vi "HolonomicController_Example.vi"(6 "EnableClosedLoop":bool=TRUE, 7 "Orientation Dmd In":dbl, 8 "Init":bool=TRUE, 9 "Reverse":bool, 10 "Follow Orientation":bool) -> (0 "AtReference":bool, 3 "Chassis Velocity Target":T2 {"vOmega" format="%10.3f"; "vY" format="%10.3f"; "vX" format="%10.3f"}, 4 "Time Offset":dbl=-1.0 format="%16.4f", 5 "Orientation Target":dbl, 11 "Gyro Heading":dbl)   [LabVIEW 2019]
uses:
  <vilib>/Rock Robotics/WPI/ThirdParty/JAS_Junk/TrajLib/TypeDef/CHASSIS_SPEEDS.ctl
  <vilib>/Rock Robotics/WPI/ThirdParty/JAS_Junk/TrajLib/TypeDef/TRAJ_STATE.ctl
  <vilib>/Rock Robotics/WPI/ThirdParty/JAS_Junk/TrajLib/TypeDef/POSE2D.ctl
  <vilib>/Rock Robotics/WPI/ThirdParty/JAS_Junk/TrajLib/TypeDef/TRANSLATION2D.ctl
  <vilib>/Rock Robotics/WPI/ThirdParty/JAS_Junk/TrajLib/TypeDef/ROTATION2D.ctl
  <vilib>/Rock Robotics/WPI/ThirdParty/JAS_Junk/TrajLib/MedianFilter_New.vi
  <vilib>/Rock Robotics/WPI/ThirdParty/JAS_Junk/TrajLib/MedianFilter_ResetToValue.vi
  SubVI/HOL_Robot Global Data.vi
  <vilib>/Rock Robotics/WPI/ThirdParty/JAS_Junk/TrajLib/MedianFilter_Calculate.vi
  <vilib>/Rock Robotics/WPI/ThirdParty/JAS_Junk/TrajLib/Trajectory_Library.lvlib
panel:
  in  "Tab Control":T1(tab)
  out "OutputTRAJ_STATE":T3={"TimeSeconds"=0.0, "Velocity"=0.0, "Acceleration"=0.0, "POSE"={"TRANSLATION"={"X"=0.0, "Y"=0.0}, "ROTATION"={"VALUE"=0.0, "COS"=1.0, "SIN"=0.0}}, "Curvature"=0.0} {"POSE"."ROTATION"."SIN" format="%13.4f"; "POSE"."ROTATION"."COS" format="%13.4f"; "POSE"."ROTATION"."VALUE" format="%13.4f"; "POSE"."TRANSLATION"."Y" format="%14.3f"; "POSE"."TRANSLATION"."X" format="%14.3f"}
  in  "Step":bool
  in  "Trajectory File Name":path=path "Sample-Robot-2-Trajectory-TrajLibrary.csv"
  out "Traj File Good":bool
  out "Module Ang\nRadians":dbl
  out "Module Speed\nM/S":dbl
  in  "Run":bool
  out "Rel Odom":T4={"TRANSLATION"={"X"=0.0, "Y"=0.0}, "ROTATION"={"VALUE"=0.0, "COS"=1.0, "SIN"=0.0}} {"ROTATION"."SIN" format="%13.4f"; "ROTATION"."COS" format="%13.4f"; "ROTATION"."VALUE" format="%13.4f"; "TRANSLATION"."Y" format="%14.3f"; "TRANSLATION"."X" format="%14.3f"}
  out "Error and Corr":T7 {"Error Pose"."ROTATION"."SIN" format="%13.4f"; "Error Pose"."ROTATION"."COS" format="%13.4f"; "Error Pose"."ROTATION"."VALUE" format="%13.4f"; "Error Pose"."TRANSLATION"."Y" format="%14.3f"; "Error Pose"."TRANSLATION"."X" format="%14.3f"}
  out "Abs Odom":T4={"TRANSLATION"={"X"=0.0, "Y"=0.0}, "ROTATION"={"VALUE"=0.0, "COS"=1.0, "SIN"=0.0}} {"ROTATION"."SIN" format="%13.4f"; "ROTATION"."COS" format="%13.4f"; "ROTATION"."VALUE" format="%13.4f"; "TRANSLATION"."Y" format="%14.3f"; "TRANSLATION"."X" format="%14.3f"}
  out "Traj Err":cluster{"X":dbl, "Y":dbl, "Angle":dbl}(graph)
  out "ChasisSpeedOutput":cluster{"vX":dbl, "vY":dbl, "vOmega":dbl}(graph)
  out "Robot Position":cluster{dbl[], dbl[]}[](graph)
  # "Module States"
  # "For now all modules use this value..."
  # "(FOR TESTING)"
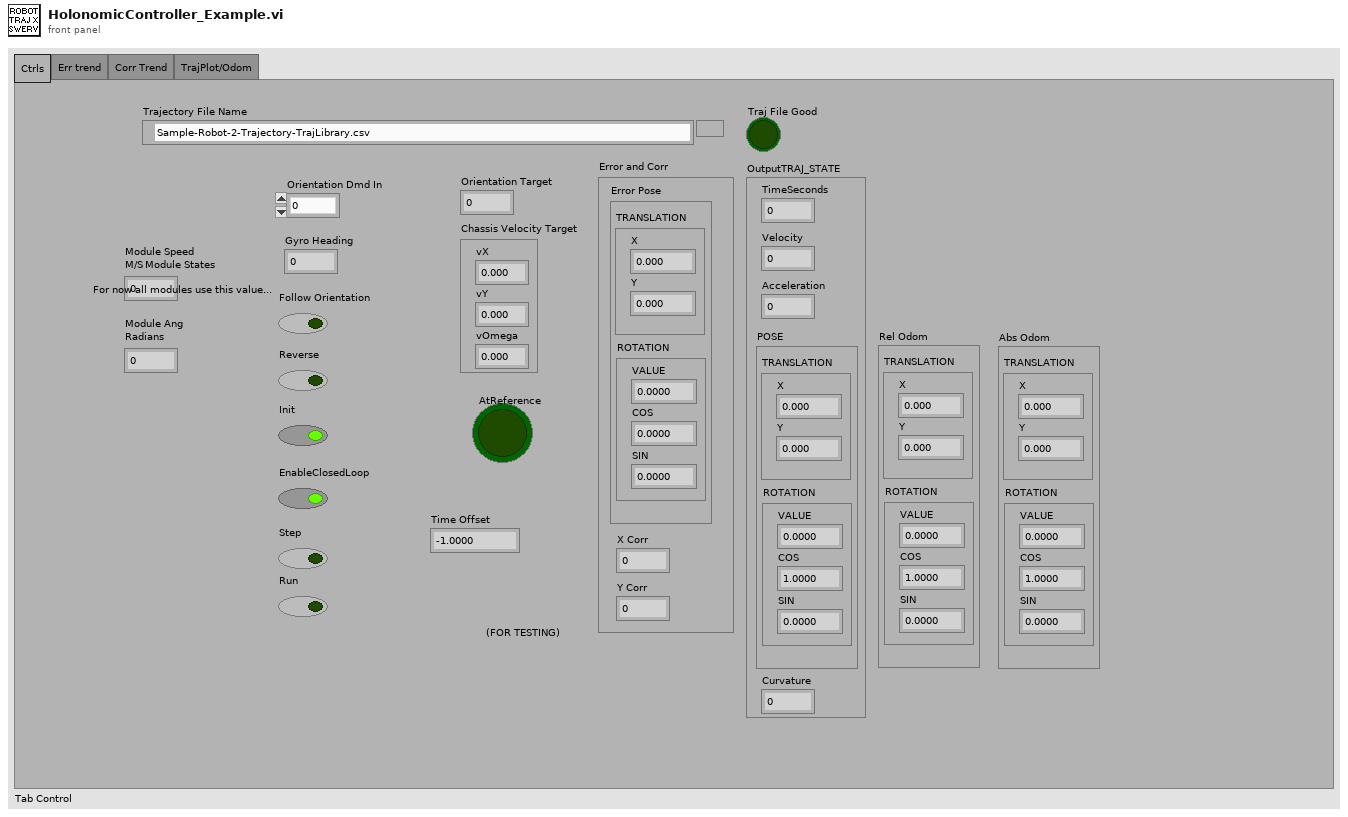
[diagram p1: front panel]
types:
  T1 = enum32{"Ctrls", "Err trend", "Corr Trend", "TrajPlot/Odom"}
  T2 = typedef "Trajectory_Library.lvlib/CHASSIS_SPEEDS.ctl" = cluster{"vX":dbl, "vY":dbl, "vOmega":dbl}
  T3 = typedef "Trajectory_Library.lvlib/TRAJ_STATE.ctl" = cluster{"TimeSeconds":dbl, "Velocity":dbl, "Acceleration":dbl, "POSE":T4, "Curvature":dbl}
  T4 = typedef "Trajectory_Library.lvlib/POSE2D.ctl" = cluster{"TRANSLATION":T5, "ROTATION":T6}
  T5 = typedef "Trajectory_Library.lvlib/TRANSLATION2D.ctl" = cluster{"X":dbl, "Y":dbl}
  T6 = typedef "Trajectory_Library.lvlib/ROTATION2D.ctl" = cluster{"VALUE":dbl, "COS":dbl, "SIN":dbl}
  T7 = cluster{"Error Pose":T4, "X Corr":dbl, "Y Corr":dbl}
  T8 = typedef "Trajectory_Library.lvlib/SWERVE_DRIVE_MODULE_POSITION.ctl" = cluster{"Distance":dbl, "Angle":T6, "P":bool}
  T9 = typedef "Trajectory_Library.lvlib/SWERVE_DRIVE_ODOMETRY.ctl" = cluster{"POSE":T4, "GyroOffset":T6, "PreviousAngle":T6, "PrevModulePositions":T8[], "NumModules":i32}
  T10 = typedef "Trajectory_Library.lvlib/SWERVE_DRIVE_KINEMATICS.ctl" = cluster{"NumModules":i32, "InverseKinematics":T11, "ForwardKinematics":T11, "Modules":T5[], "PrevCoR":T5, "SavedModuleStates":T12[]}
  T11 = typedef "NI_Matrix.lvlib/RealMatrix.ctl" = dbl[][]
  T12 = typedef "Trajectory_Library.lvlib/SWERVE_DRIVE_MODULE_STATE.ctl" = cluster{"Speed":dbl, "Angle":T6}
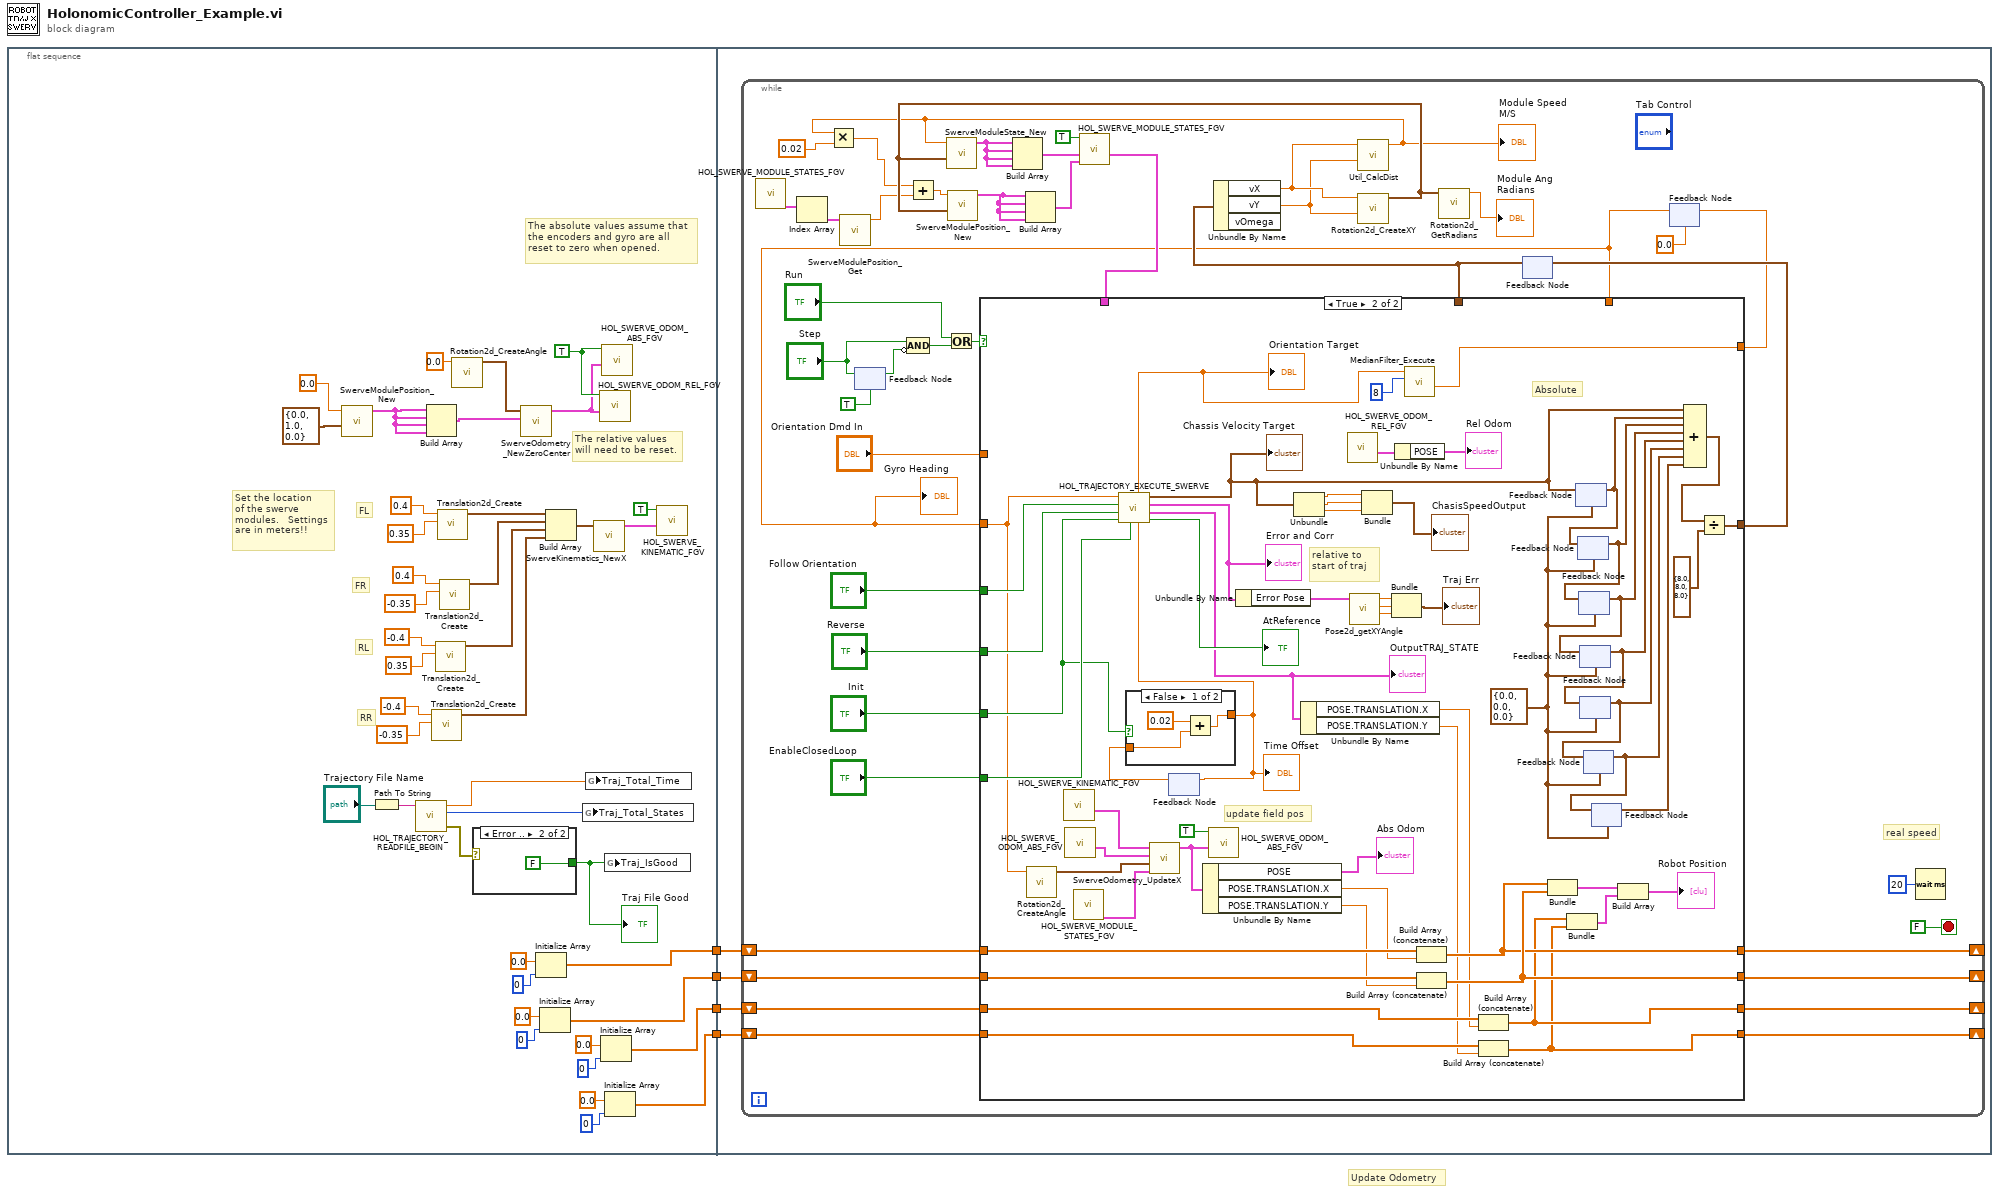
[diagram p0: block diagram]
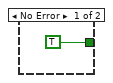
[diagram p2: hidden frame]
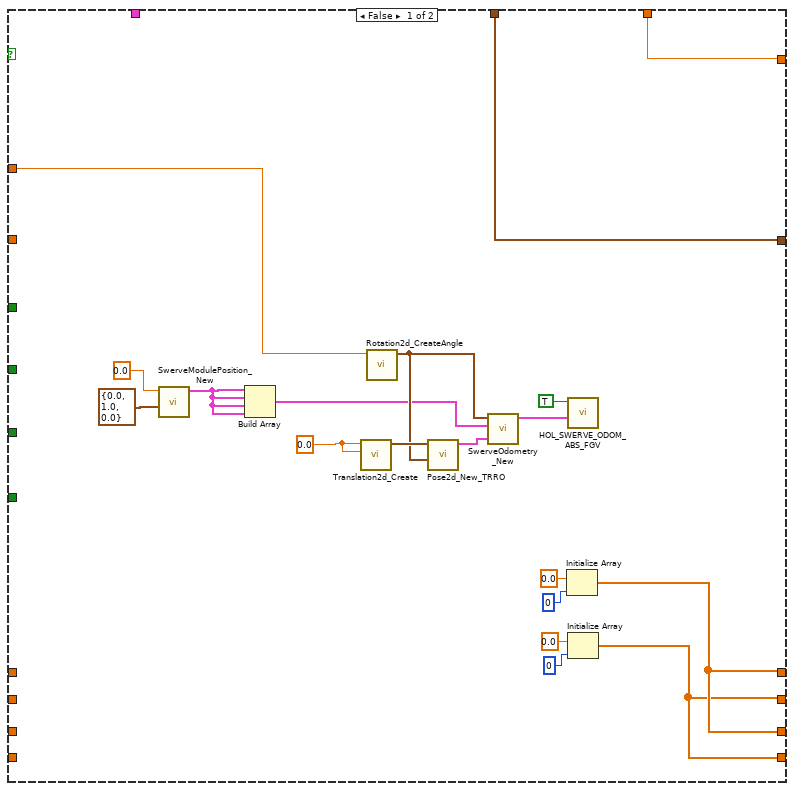
[diagram p3: hidden frame]
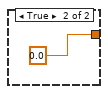
[diagram p4: hidden frame]
diagram:
  # "Update Odometry"
  n1 = flat-sequence {
    tunnel: [w20] -> w4
    tunnel: [w17] -> w3
    tunnel: [w6] -> w2
    tunnel: [w5] -> w1
    tunnel: w4 -> [w51]
    tunnel: w3 -> [w50]
    tunnel: w2 -> [w49]
    tunnel: w1 -> [w48]
    frame #0 {
      w16 = TRUE ("WRITE")
      # "The absolute values assume that\nthe encoders and gyro are all\nreset to zero when opened."
      # "RR"
      # "RL"
      # "FR"
      # "FL"
      # "Set the location\nof the swerve \nmodules.   Settings\nare in meters!!"
      # "The relative values\nwill need to be reset."
      n2 = call <vilib>:"SwerveModulePosition_New.vi"("ROTATION"=T6 {"VALUE"=0.0, "COS"=1.0, "SIN"=0.0}, "Distance"=0.0) -> ("SWERVE_DRIVE_MODULE_POSITION"=w12:T8)  [unwired: 9 in]
      n3 = Path To String(path="Trajectory File Name") -> (string=w42:string)
      n4 = call "HOL_TRAJECTORY_READFILE_BEGIN.vi"("Trajectory File Name"=w42) -> ("error out"=w45:errorcluster, "Trajectory Items"=w43:i32, "TotalTImeSecs"=w44:dbl)  [unwired: 8 in]
      n5 = Build Array(w12, w12, w12, w12) -> (w11:T8[])
      n6 = call <vilib>:"Translation2d_Create.vi"("Y"=-0.35, "X"=-0.4) -> ("TRANSLATION"=w23:T5)  [unwired: 9 in]
      n7 = call <vilib>:"Translation2d_Create.vi"("Y"=0.35, "X"=-0.4) -> ("TRANSLATION"=w29:T5)  [unwired: 9 in]
      n8 = call <vilib>:"Translation2d_Create.vi"("Y"=0.35, "X"=0.4) -> ("TRANSLATION"=w31:T5)  [unwired: 9 in]
      n9 = call <vilib>:"Translation2d_Create.vi"("Y"=-0.35, "X"=0.4) -> ("TRANSLATION"=w30:T5)  [unwired: 9 in]
      n10 = call <vilib>:"Rotation2d_CreateAngle.vi"("Angle"=0.0) -> ("ROTATION"=w38:T6)  [unwired: 10 in]
      n11 = case shown="Error .." w45 {
        tunnel: [TRUE FALSE] -> w40
        frame No Error {
        }
        frame Error {
        }
      }
      "Traj File Good" <- w40
      n12 = call <vilib>:"SwerveOdometry_NewZeroCenter.vi"("Module Positions"=w11, "gyroAngle"=w38) -> ("SWERVE_DRIVE_ODOMETRY"=w15:T9)  [unwired: 9 in]
      n13 = Initialize Array(0.0 ("element"), 0 ("dimension size")) -> (w20:dbl[])
      n14 = Initialize Array(0.0 ("element"), 0 ("dimension size")) -> (w17:dbl[])
      n15 = Build Array(w31, w30, w29, w23) -> (w28:T5[])
      n16 = global write "HOL_Robot Global Data.vi" "Traj_Total_States"(w43) -> ()
      n17 = global write "HOL_Robot Global Data.vi" "Traj_Total_Time"(w44) -> ()
      n18 = call <vilib>:"SwerveKinematics_NewX.vi"("Wheels"=w28) -> ("SWERVE_DRIVE_KINEMATICS"=w26:T10)  [unwired: 10 in]
      n19 = call "HOL_SWERVE_ODOM_REL_FGV.vi"("in SWERVE_DRIVE_ODOMETRY"=w15, "WRITE"=w16) -> ()  [unwired: 9 in, 1 out]
      n20 = Initialize Array(0.0 ("element"), 0 ("dimension size")) -> (w6:dbl[])
      n21 = call "HOL_SWERVE_ODOM_ABS_FGV.vi"("in SWERVE_DRIVE_ODOMETRY"=w15, "WRITE"=w16) -> ()  [unwired: 9 in, 1 out]
      n22 = global write "HOL_Robot Global Data.vi" "Traj_IsGood"(w40) -> ()
      n23 = Initialize Array(0.0 ("element"), 0 ("dimension size")) -> (w5:dbl[])
      n24 = call "HOL_SWERVE_KINEMATIC_FGV.vi"("in SWERVE_DRIVE_KINEMATICS"=w26, "WRITE"=TRUE) -> ()  [unwired: 9 in, 1 out]
    }
    frame #1 {
      n25 = while {
        shift-right: [w66] -> _
        shift-left: w51 -> [w69]
        shift-right: [w67] -> _
        shift-left: w50 -> [w68]
        shift-right: [w55] -> _
        shift-left: w49 -> [w53]
        shift-right: [w54] -> _
        shift-left: w48 -> [w52]
        stop <- FALSE stop-if-true
        # "real speed"
        n26 = call "HOL_SWERVE_MODULE_STATES_FGV.vi"() -> ("Out Current Module Positions"=w63:T8[])  [unwired: 10 in, 1 out]
        n27 = Index Array(array=w63) -> (element=w62:T8)  [unwired: 1 in]
        n28 = call <vilib>:"SwerveModulePosition_Get.vi"("Swerve Module Position"=w62) -> ("Distance M"=w56:dbl)  [unwired: 8 in, 2 out]
        n29 = feedback #1(TRUE ("Step")) -> (w91:bool)
        n30 = feedback-in #1("Step") -> ()
        n31 = Compound Arithmetic op=AND("Step", invert w91) -> (w76:bool)
        n32 = Or(x="Run", y=w76) -> (x .or. y?=w75:bool)
        n33 = feedback #2() -> (w80:T2)  [unwired: 1 in]
        n34 = Unbundle By Name(w80) -> ("vX"=w79:dbl, "vY"=w78:dbl)  [unwired: 1 out]
        n35 = call <vilib>:"Util_CalcDist.vi"("Y"=w78, "X"=w79) -> ("DIST"=w60:dbl)  [unwired: 9 in]
        "Module Speed\nM/S" <- w60
        n36 = Multiply(x=w60, y=0.02) -> (x*y=w57:dbl)
        n37 = Add(x=w57, y=w56) -> (x+y=w58:dbl)
        n38 = call <vilib>:"Rotation2d_CreateXY.vi"("Y or sine"=w78, "X or  cosine"=w79) -> ("ROTATION"=w61:T6)  [unwired: 9 in]
        n39 = call <vilib>:"SwerveModuleState_New.vi"("ROTATION"=w61, "Speed"=w60) -> ("SWERVE_DRIVE_MODULE_STATE"=w83:T12)  [unwired: 9 in]
        n40 = call <vilib>:"SwerveModulePosition_New.vi"("ROTATION"=w61, "Distance"=w58) -> ("SWERVE_DRIVE_MODULE_POSITION"=w65:T8)  [unwired: 9 in]
        n41 = Build Array(w83, w83, w83, w83) -> (w84:T12[])
        n42 = Build Array(w65, w65, w65, w65) -> (w64:T8[])
        n43 = call "HOL_SWERVE_MODULE_STATES_FGV.vi"("in Current Module Positions"=w64, "in Current Module States"=w84, "WRITE"=TRUE) -> ("out Current Module States"=w85:T12[])  [unwired: 7 in, 1 out]
        n44 = call <vilib>:"Rotation2d_GetRadians.vi"("in ROTATION"=w61) -> ("AngleRadians"=→"Module Ang\nRadians":dbl)  [unwired: 10 in]
        n45 = feedback #3(0.0 ("MedianValue")) -> (w71:dbl)
        "Gyro Heading" <- w71
        n46 = case shown="True" w75 {
          tunnel: w71 -> [_ w134]
          tunnel: "Follow Orientation" -> [_ w171]
          tunnel: "Reverse" -> [_ w170]
          tunnel: "Init" -> [_ w166]
          tunnel: "EnableClosedLoop" -> [_ w169]
          tunnel: "Orientation Dmd In" -> [w106 _]
          tunnel: w85 -> [_ _]
          tunnel: [w113 w154] -> w81
          tunnel: w80 -> [w113 _]
          tunnel: [w112 w147] -> w73
          tunnel: w71 -> [w112 _]
          tunnel: w69 -> [_ w141]
          tunnel: w68 -> [_ w142]
          tunnel: [w95 w140] -> w67
          tunnel: [w96 w139] -> w66
          tunnel: [w96 w118] -> w55
          tunnel: [w95 w117] -> w54
          tunnel: w53 -> [_ w122]
          tunnel: w52 -> [_ w120]
          frame False {
            w104 = 0.0 ("X")
            n47 = call <vilib>:"SwerveModulePosition_New.vi"("ROTATION"=T6 {"VALUE"=0.0, "COS"=1.0, "SIN"=0.0}, "Distance"=0.0) -> ("SWERVE_DRIVE_MODULE_POSITION"=w99:T8)  [unwired: 9 in]
            n48 = Build Array(w99, w99, w99, w99) -> (w98:T8[])
            n49 = call <vilib>:"Translation2d_Create.vi"("Y"=w104, "X"=w104) -> ("TRANSLATION"=w105:T5)  [unwired: 9 in]
            n50 = call <vilib>:"Rotation2d_CreateAngle.vi"("Angle"=w106) -> ("ROTATION"=w103:T6)  [unwired: 10 in]
            n51 = call <vilib>:"Pose2d_New_TRRO.vi"("ROTATION"=w103, "TRANSLATION"=w105) -> ("outPOSE"=w102:T4)  [unwired: 9 in]
            n52 = call <vilib>:"SwerveOdometry_New.vi"("InitialPose"=w102, "Module Positions"=w98, "gyroAngle"=w103) -> ("SWERVE_DRIVE_ODOMETRY"=w101:T9)  [unwired: 8 in]
            n53 = Initialize Array(0.0 ("element"), 0 ("dimension size")) -> (w96:dbl[])
            n54 = call "HOL_SWERVE_ODOM_ABS_FGV.vi"("in SWERVE_DRIVE_ODOMETRY"=w101, "WRITE"=TRUE) -> ()  [unwired: 9 in, 1 out]
            n55 = Initialize Array(0.0 ("element"), 0 ("dimension size")) -> (w95:dbl[])
          }
          frame True {
            w164 = T2 {"vX"=0.0, "vY"=0.0, "vOmega"=0.0} ("Chassis Velocity Target")
            # "update field pos"
            # "Absolute"
            # "relative to start of traj"
            n56 = call <vilib>:"Rotation2d_CreateAngle.vi"("Angle"=w134) -> ("ROTATION"=w127:T6)  [unwired: 10 in]
            n57 = call "HOL_SWERVE_KINEMATIC_FGV.vi"() -> ("out SWERVE_DRIVE_KINEMATICS"=w125:T10)  [unwired: 11 in]
            n58 = call "HOL_SWERVE_ODOM_ABS_FGV.vi"() -> ("out SWERVE_DRIVE_ODOMETRY"=w126:T9)  [unwired: 11 in]
            n59 = call "HOL_SWERVE_MODULE_STATES_FGV.vi"() -> ("Out Current Module Positions"=w124:T8[])  [unwired: 10 in, 1 out]
            n60 = call <vilib>:"SwerveOdometry_UpdateX.vi"("module Positions"=w124, "gyroAngle"=w127, "in SWERVE_DRIVE_ODOMETRY"=w126, "SWERVE_DRIVE_KINEMATICS"=w125) -> ("out SWERVE_DRIVE_ODOMETRY"=w137:T9)  [unwired: 5 in, 2 out]
            n61 = feedback #4() -> (w167:dbl)  [unwired: 1 in]
            n62 = case shown="False" w166 {
              tunnel: [w174 0.0] -> w165
              tunnel: w167 -> [w172 _]
              frame False {
                n63 = Add(x=0.02, y=w172) -> (x+y=w174:dbl)
              }
              frame True {
              }
            }
            "Time Offset" <- w165
            n64 = call "HOL_TRAJECTORY_EXECUTE_SWERVE.vi"("Time Offset"=w165, "EnableClosedLoop"=w169, "Init"=w166, "Reverse"=w170, "Follow Orientation"=w171, "Gyro Heading\nRAD"=w134) -> ("AtReference"=→"AtReference":bool, "OutputTRAJ_STATE"=w123:T3, "Error and Corr"=w146:T7, "Chassis Velocity Target"=w132:T2, "Orientation Target"=w149:dbl)  [unwired: 1 in]
            "Orientation Target" <- w149
            "Chassis Velocity Target" <- w132
            "OutputTRAJ_STATE" <- w123
            "Error and Corr" <- w146
            n65 = feedback-in #4(w165) -> ()
            n66 = Unbundle By Name(w137) -> ("POSE"=→"Abs Odom":T4, "POSE.TRANSLATION.X"=w136:dbl, "POSE.TRANSLATION.Y"=w135:dbl)
            n67 = call "HOL_SWERVE_ODOM_ABS_FGV.vi"("in SWERVE_DRIVE_ODOMETRY"=w137, "WRITE"=TRUE) -> ()  [unwired: 9 in, 1 out]
            n68 = Unbundle By Name(w146) -> ("Error Pose"=w145:T4)
            n69 = Unbundle(w132) -> ("vX"=w130:dbl, "vY"=w129:dbl, "vOmega"=w128:dbl)
            n70 = Unbundle By Name(w123) -> ("POSE.TRANSLATION.X"=w121:dbl, "POSE.TRANSLATION.Y"=w119:dbl)
            n71 = call "HOL_SWERVE_ODOM_REL_FGV.vi"() -> ("out SWERVE_DRIVE_ODOMETRY"=w143:T9)  [unwired: 11 in]
            n72 = call <vilib>:"Pose2d_getXYAngle.vi"("in POSE"=w145) -> ("Angle"=w150:dbl, "Y"=w151:dbl, "X"=w152:dbl)  [unwired: 8 in]
            n73 = Bundle("vX"=w130, "vY"=w129, "vOmega"=w128) -> (→"ChasisSpeedOutput":cluster{"vX":dbl, "vY":dbl, "vOmega":dbl})  [unwired: 1 in]
            n74 = Bundle("X"=w152, "Y"=w151, "Angle"=w150) -> (→"Traj Err":cluster{"X":dbl, "Y":dbl, "Angle":dbl})  [unwired: 1 in]
            n75 = Unbundle By Name(w143) -> ("POSE"=→"Rel Odom":T4)
            n76 = call <vilib>:"MedianFilter_Execute.vi"("Samples"=8, "Input Value"=w149) -> ("MedianValue"=w147:dbl)  [unwired: 8 in, 1 out]
            n77 = Build Array (concatenate)(w141, w136) -> (w139:dbl[])
            n78 = Build Array (concatenate)(w142, w135) -> (w140:dbl[])
            n79 = Build Array (concatenate)(w122, w121) -> (w118:dbl[])
            n80 = Build Array (concatenate)(w120, w119) -> (w117:dbl[])
            n81 = Bundle(w139, w140) -> (w116:cluster{dbl[], dbl[]})  [unwired: 1 in]
            n82 = Bundle(w118, w117) -> (w115:cluster{dbl[], dbl[]})  [unwired: 1 in]
            n83 = feedback-in #5(w132) -> ()
            n84 = feedback #5(w164) -> (w163:T2)
            n85 = feedback #6(w164) -> (w162:T2)
            n86 = feedback-in #6(w163) -> ()
            n87 = feedback #7(w164) -> (w161:T2)
            n88 = feedback-in #7(w162) -> ()
            n89 = feedback #8(w164) -> (w160:T2)
            n90 = feedback-in #8(w161) -> ()
            n91 = feedback #9(w164) -> (w159:T2)
            n92 = feedback-in #9(w160) -> ()
            n93 = feedback #10(w164) -> (w158:T2)
            n94 = feedback-in #10(w159) -> ()
            n95 = feedback #11(w164) -> (w157:T2)
            n96 = feedback-in #11(w158) -> ()
            n97 = Build Array(w116, w115) -> (→"Robot Position":cluster{dbl[], dbl[]}[])
            n98 = Compound Arithmetic op=ADD(w132, w163, w162, w161, w160, w159, w158, w157) -> (w156:T2)
            n99 = Divide(x=w156, y=T2 {"vX"=8.0, "vY"=8.0, "vOmega"=8.0}) -> (x/y=w154:T2)
          }
        }
        n100 = feedback-in #2(w81) -> ()
        n101 = feedback-in #3(w73) -> ()
        n102 = Wait (ms)(milliseconds to wait=u32 20) -> ()  [unwired: 1 out]
      }
    }
  }
